vi "all-signals+drivingtorque-v-aacc-n_motor.vi"() -> ()   [LabVIEW 2018]
uses:
  <vilib>/Analysis/baseanly.llb/Mean (DBL).vi
  <vilib>/Analysis/NI_AALBase.lvlib
panel:
  out "duplicate waveform":waveform(dbl)(graph)
  out "driving torque":dynamicdata(graph)
  out "XY Graph 2":cluster{"Y":dbl[], "Y":dbl[]}[](graph)
  out "Motordrehzahl":dynamicdata(graph)
  out "RPM and dn":dynamicdata(graph)
  in  "stop driving torque":bool
  out "angular acc":dynamicdata(graph)
  in  "Clear Charts":bool
  in  "stop clear charts":bool
  in  "stop  counter (F)":bool caption="counter stop (F)"
  in  "stop I,U,M_brems (F)":bool caption="IU P STOP (F)"
  out "Driving Torque gemittelt":dbl(graph)
  out "RPM":dbl
  in  "Messzeit in ms":u32=100 min=10 max=1000 step=10
  out "Bremsmoment":dynamicdata(graph)
  out "Strom, Spannung, elektrische Leistung":dynamicdata(graph)
  out "Geschwindigkeit":dynamicdata(graph)
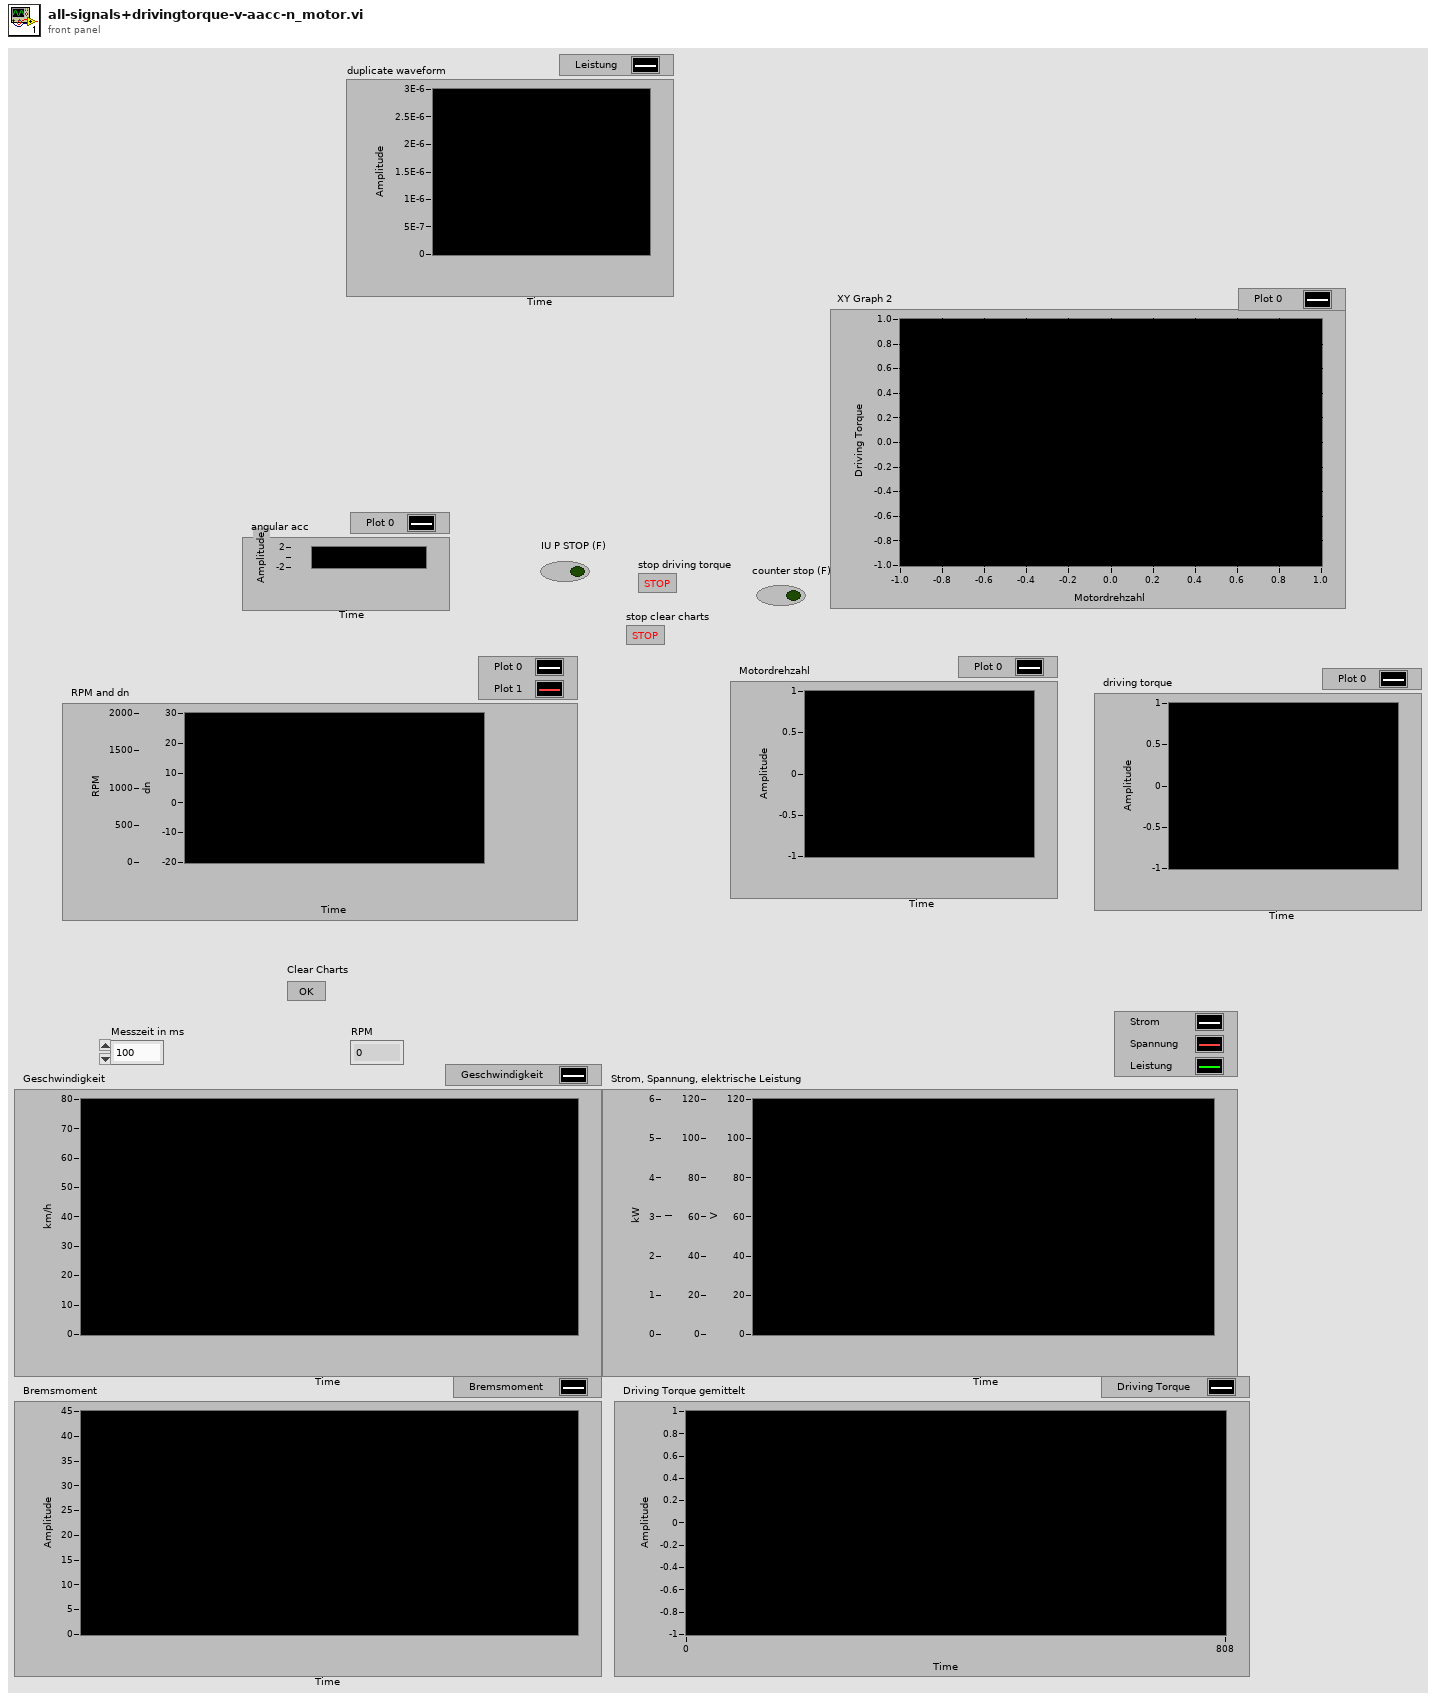
[diagram p1: front panel]
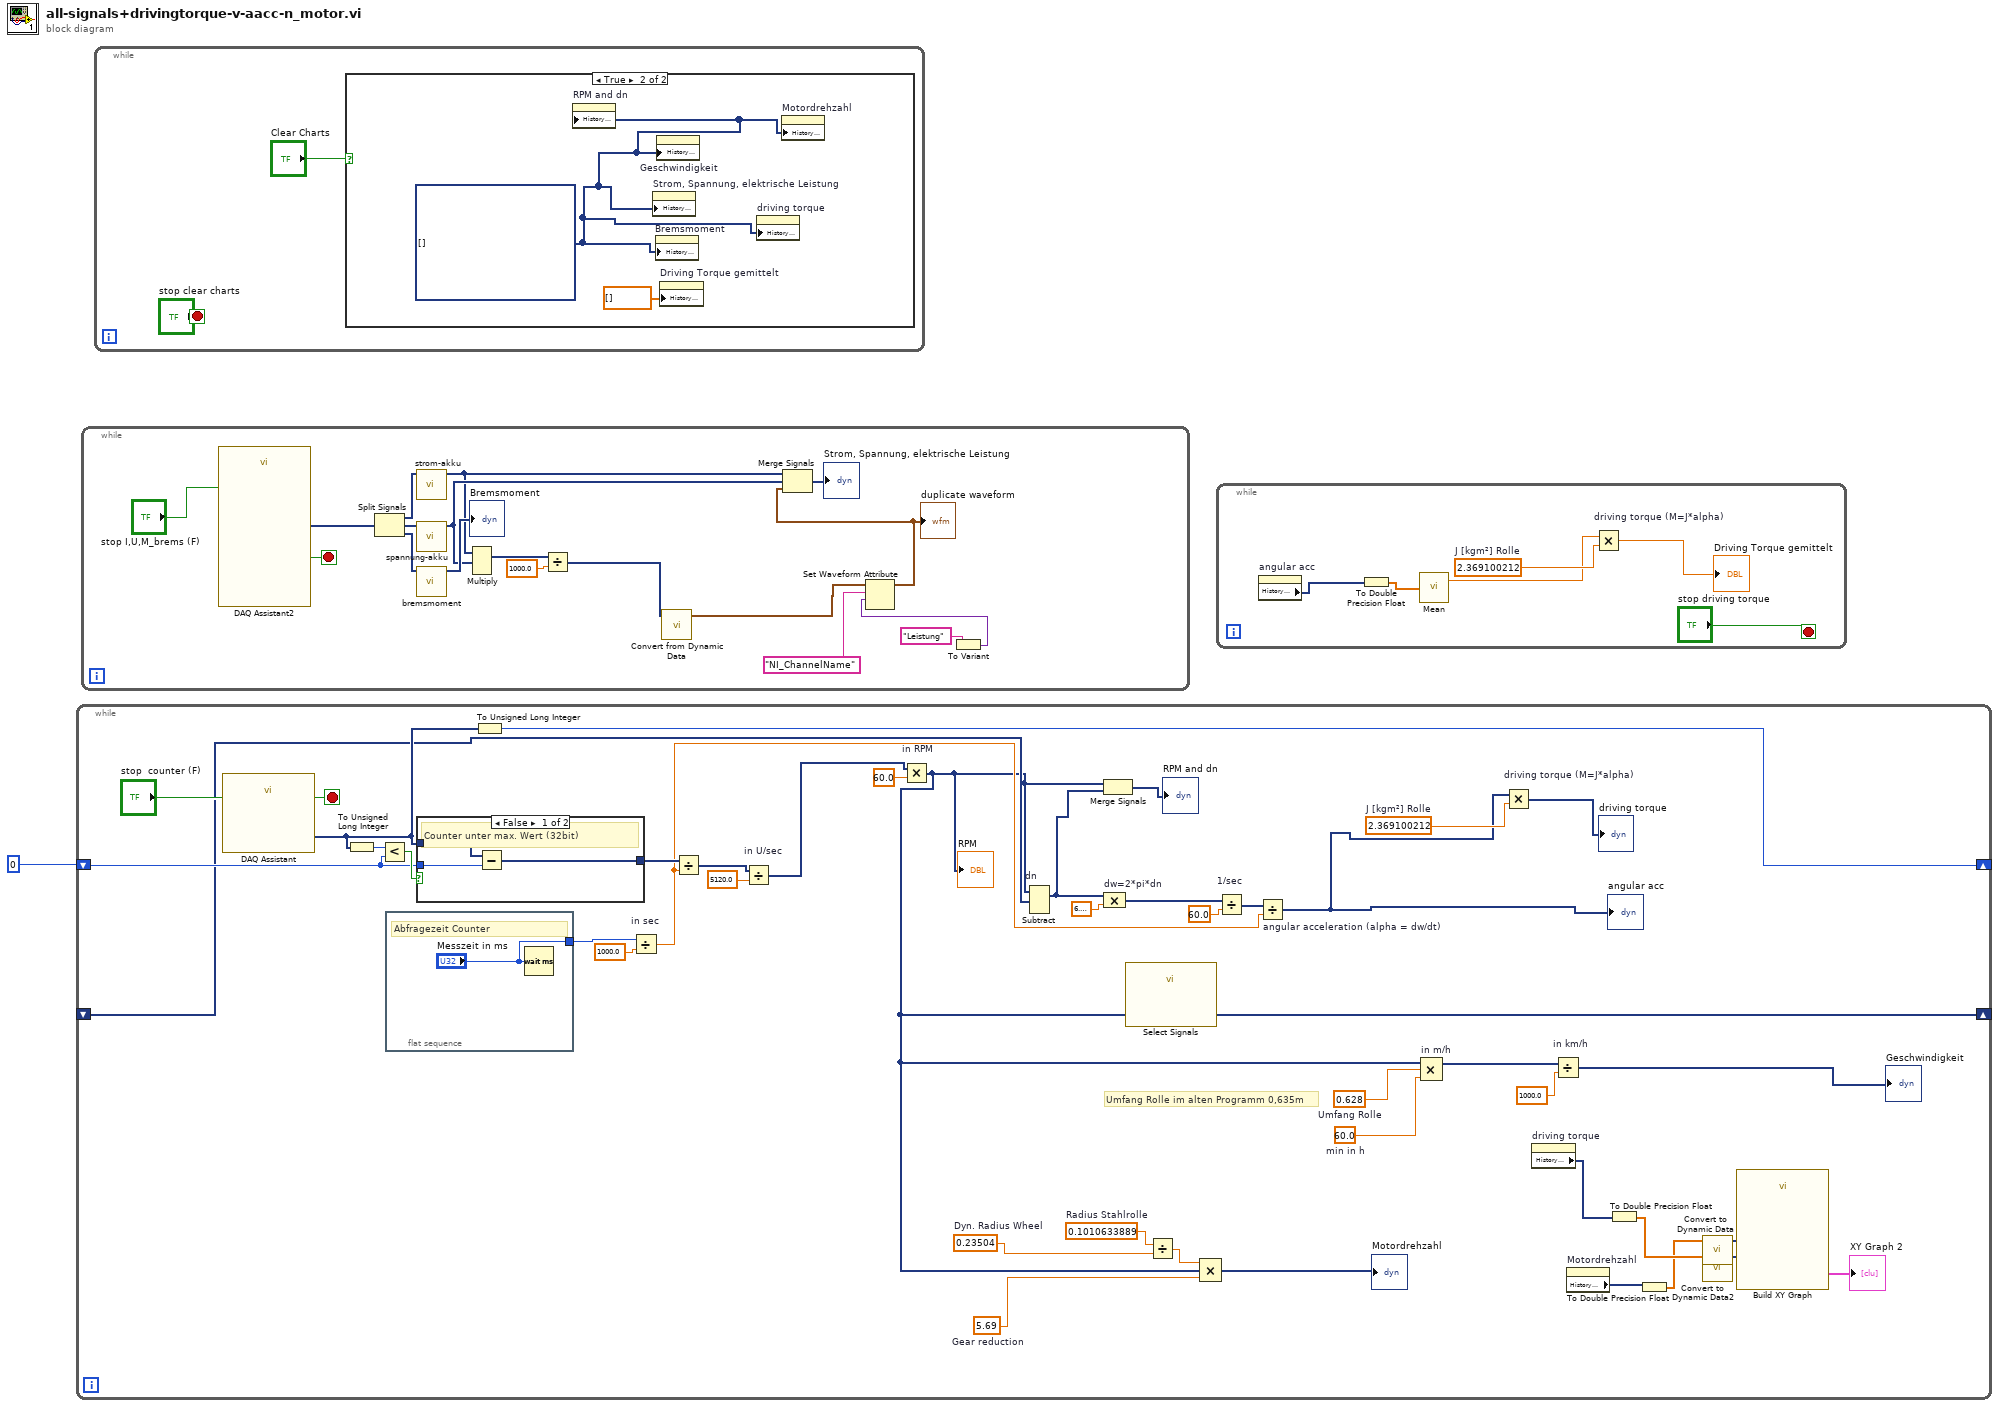
[diagram p0: block diagram]
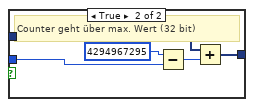
[diagram p2: hidden frame]
diagram:
  n1 = while {
    shift-right: [w42] -> _
    shift-left: u32 0 -> [w21]
    shift-right: [w15] -> _
    shift-left: _ -> [w19]
    stop <- w40 stop-if-true
    w11 = 2.369100212  # J [kgm²] Rolle
    w13 = 5.69  # Gear reduction
    w14 = 0.23504  # Dyn. Radius Wheel
    w17 = 0.1010633889  # Radius Stahlrolle
    w27 = 60.0  # min in h
    w26 = 0.628  # Umfang Rolle
    # "Umfang Rolle im alten Programm 0,635m"
    n2 = call "DAQ Assistant"("stop (F)"="stop  counter (F)") -> ("data"=w22:dynamicdata, "stopped"=w40:bool)  [unwired: 15 in, 2 out]
    n3 = To Unsigned Long Integer(number=w22) -> (unsigned 32bit integer=w41:u32)
    n4 = Less?(x=w41, y=w21) -> (x < y?=w44:bool)
    n5 = flat-sequence {
      tunnel: ["Messzeit in ms"] -> w39
      frame #0 {
        # "Abfragezeit Counter"
        n6 = Wait (ms)(milliseconds to wait="Messzeit in ms") -> ()  [unwired: 1 out]
      }
    }
    n7 = case shown="False" w44 {
      tunnel: w22 -> [w48 w50]
      tunnel: w21 -> [w47 w52]
      tunnel: [w46 w49] -> w37
      frame False {
        # "Counter unter max. Wert (32bit)"
        n8 = Subtract(x=w48, y=w47) -> (x-y=w46:dynamicdata)
      }
      frame True {
        # "Counter geht über max. Wert (32 bit)"
        n9 = Subtract(x=u32 4294967295, y=w52) -> (x-y=w51:u32)
        n10 = Add(x=w50, y=w51) -> (x+y=w49:dynamicdata)
      }
    }
    n11 = To Unsigned Long Integer(number=w22) -> (unsigned 32bit integer=w42:u32)
    n12 = Divide "in sec"(x=w39, y=1000.0) -> (x/y=w30:dbl)
    n13 = Divide(x=w37, y=w30) -> (x/y=w36:dynamicdata)
    n14 = Divide "in U/sec"(x=w36, y=5120.0) -> (x/y=w24:dynamicdata)
    n15 = Multiply "in RPM"(x=w24, y=60.0) -> (x*y=w15:dynamicdata)
    "RPM" <- w15
    n16 = Subtract "dn"(1:w19, 2:w15) -> (0:w18:dynamicdata)  [unwired: 1 in, 1 out]
    n17 = Merge Signals(w15, w18) -> (→"RPM and dn":dynamicdata)
    n18 = Compound Arithmetic op=MULTIPLY "dw=2*pi*dn"(w18, 6.283185307179586) -> (w33:dynamicdata)
    n19 = call "Select Signals"() -> ()  [unwired: 10 in, 2 out]
    n20 = Divide(x=w17, y=w14) -> (x/y=w16:dbl)
    n21 = Compound Arithmetic op=MULTIPLY(w16, w15, w13) -> (→"Motordrehzahl":dynamicdata)
    n22 = Divide "1/sec"(x=w33, y=60.0) -> (x/y=w31:dynamicdata)
    n23 = Divide "angular acceleration (alpha = dw/dt)"(x=w31, y=w30) -> (x/y=w2:dynamicdata)
    "angular acc" <- w2
    n24 = Compound Arithmetic op=MULTIPLY "in m/h"(w15, w26, w27) -> (w28:dynamicdata)
    n25 = Multiply "driving torque (M=J*alpha)"(x=w2, y=w11) -> (x*y=→"driving torque":dynamicdata)
    n26 = property on="driving torque" class="WFChart (strict)"() -> ("History Data"=w9:dynamicdata[])  [unwired: 2 in, 2 out]
    n27 = Divide "in km/h"(x=w28, y=1000.0) -> (x/y=→"Geschwindigkeit":dynamicdata)
    n28 = property on="Motordrehzahl" class="WFChart (strict)"() -> ("History Data"=w5:dynamicdata[])  [unwired: 2 in, 2 out]
    n29 = To Double Precision Float(number=w9) -> (double precision float=w8:dbl[])
    n30 = To Double Precision Float(number=w5) -> (double precision float=w4:dbl[])
    n31 = call "Convert to Dynamic Data"("Array"=w4) -> ("Dynamic Data Type"=w6:dynamicdata)  [unwired: 3 in]
    n32 = call "Convert to Dynamic Data2"("Array"=w8) -> ("Dynamic Data Type"=w7:dynamicdata)  [unwired: 3 in]
    n33 = call "Build XY Graph"("Y Input"=w7, "X Input"=w6) -> ("XY Graph"=→"XY Graph 2":cluster{"X":dbl[], "Y":dbl[]}[])  [unwired: 8 in, 1 out]
  }
  n34 = while {
    stop <- w65 stop-if-true
    n35 = call "DAQ Assistant2"("stop (F)"="stop I,U,M_brems (F)") -> ("data"=w66:dynamicdata, "stopped"=w65:bool)  [unwired: 15 in, 2 out]
    n36 = Split Signals(w66) -> (w71:dynamicdata, w70:dynamicdata, w69:dynamicdata)  [unwired: 3 in]
    n37 = call "strom-akku.vi"("Dynamic Data"=w71) -> ("Filtered Signal"=w63:dynamicdata)  [unwired: 10 in]
    n38 = call "spannung-akku.vi"("Dynamic Data in"=w70) -> ("Dynamic Data out"=w64:dynamicdata)  [unwired: 10 in]
    n39 = call "bremsmoment.vi"("Dynamic Data in"=w69) -> ("Dynamic Data out"=→"Bremsmoment":dynamicdata)  [unwired: 10 in]
    n40 = Multiply(1:w64, 2:w63) -> (0:w61:dynamicdata)  [unwired: 1 in, 1 out]
    n41 = Divide(x=w61, y=1000.0) -> (x/y=w59:dynamicdata)
    n42 = call "Convert from Dynamic Data"("Dynamic Data Type"=w59) -> ("Waveform"=w58:waveform(dbl))  [unwired: 3 in]
    n43 = To Variant(anything="Leistung") -> (Variant=w55:variant)
    n44 = Set Waveform Attribute(5:w55, 6:"NI_ChannelName" ("name"), 7:w58) -> (3:w54:waveform(dbl))  [unwired: 1 in, 2 out]
    "duplicate waveform" <- w54
    n45 = Merge Signals(w63, w64, w54) -> (→"Strom, Spannung, elektrische Leistung":dynamicdata)
  }
  n46 = while {
    stop <- "stop clear charts" stop-if-true
    n47 = case shown="True" "Clear Charts" {
      frame False {
      }
      frame True {
        w74 = dynamicdata[] [] ("History Data")
        n48 = property on="RPM and dn" class="WFChart (strict)"("History Data"=w74) -> ()  [unwired: 2 in, 2 out]
        n49 = property on="Strom, Spannung, elektrische Leistung" class="WFChart (strict)"("History Data"=w74) -> ()  [unwired: 2 in, 2 out]
        n50 = property on="Bremsmoment" class="WFChart (strict)"("History Data"=w74) -> ()  [unwired: 2 in, 2 out]
        n51 = property on="Geschwindigkeit" class="WFChart (strict)"("History Data"=w74) -> ()  [unwired: 2 in, 2 out]
        n52 = property on="Driving Torque gemittelt" class="WFChart (strict)"("History Data"=dbl[] []) -> ()  [unwired: 2 in, 2 out]
        n53 = property on="driving torque" class="WFChart (strict)"("History Data"=w74) -> ()  [unwired: 2 in, 2 out]
        n54 = property on="Motordrehzahl" class="WFChart (strict)"("History Data"=w74) -> ()  [unwired: 2 in, 2 out]
      }
    }
  }
  n55 = while {
    stop <- "stop driving torque" stop-if-true
    w80 = 2.369100212  # J [kgm²] Rolle
    n56 = property on="angular acc" class="WFChart (strict)"() -> ("History Data"=w76:dynamicdata[])  [unwired: 2 in, 2 out]
    n57 = To Double Precision Float(number=w76) -> (double precision float=w81:dbl[])
    n58 = call-poly <vilib>:"Mean.vi"("X"=w81) -> ("mean"=w78:dbl)  [unwired: 1 out]
    n59 = Multiply "driving torque (M=J*alpha)"(x=w78, y=w80) -> (x*y=→"Driving Torque gemittelt":dbl)
  }
